vi "Actor Core.vi"(8 "error in":errorcluster, 11 "MQTT-Server in":refnum<class "MQTT-Server.lvclass">) -> (0 "error out":errorcluster, 3 "Actor out":refnum<class "Actor.lvclass">)   [LabVIEW 2023, in "MQTT-Server.lvlib" / "MQTT-Server.lvclass"]
doc: "(<B>Filename</B>: Actor Framework.lvlib:Actor.lvclass:Actor Core.vi)\n\nReceives messages to the actor, reacts to them, and initiates any error handling that may shut the actor down.\n\nDescendant classes may override this VI to append parallel tasks for the actor to complete while it handles messages. Overrides use the Call Parent Class Method node."
uses:
  MQTT-Server.lvclass
  <vilib>/ActorFramework/Actor/Actor.lvclass
  MQTT-Server.lvclass/MQTT-Server.ctl
  <vilib>/G Open Source Project for LabVIEW/MQTT Broker/Server class/Server.lvclass
  C:/Program Files/National Instruments/LabVIEW 2023/vi.lib/LabVIEW Open Source Project/MQTT Connection/MQTT_Base/Base Class/MQTT_Base.lvclass
  <vilib>/LabVIEW Open Source Project/MQTT Connection/MQTT_Base/Base Class/MQTT_Base.lvclass
panel:
  out "Chart":waveform(dbl)[](graph)
  out "NbConnections":u32
  out "Inbound Message":string
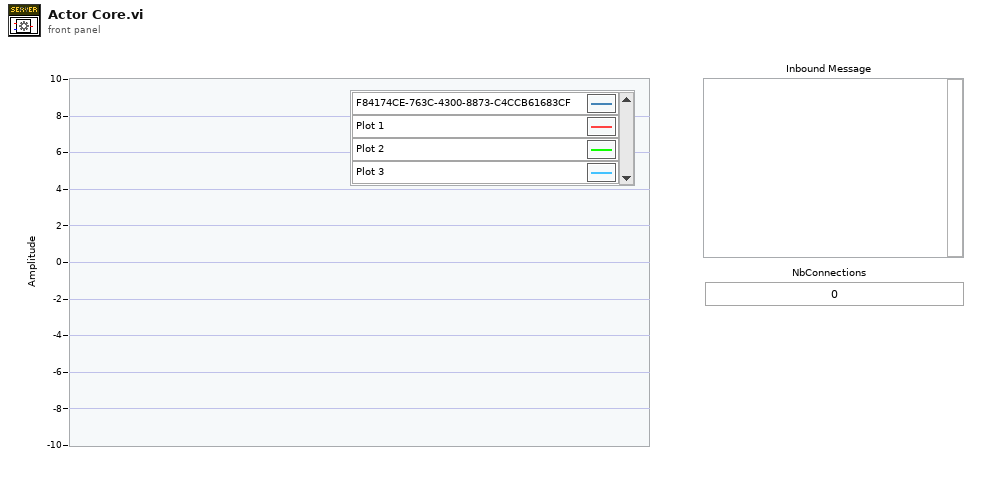
[diagram p1: front panel]
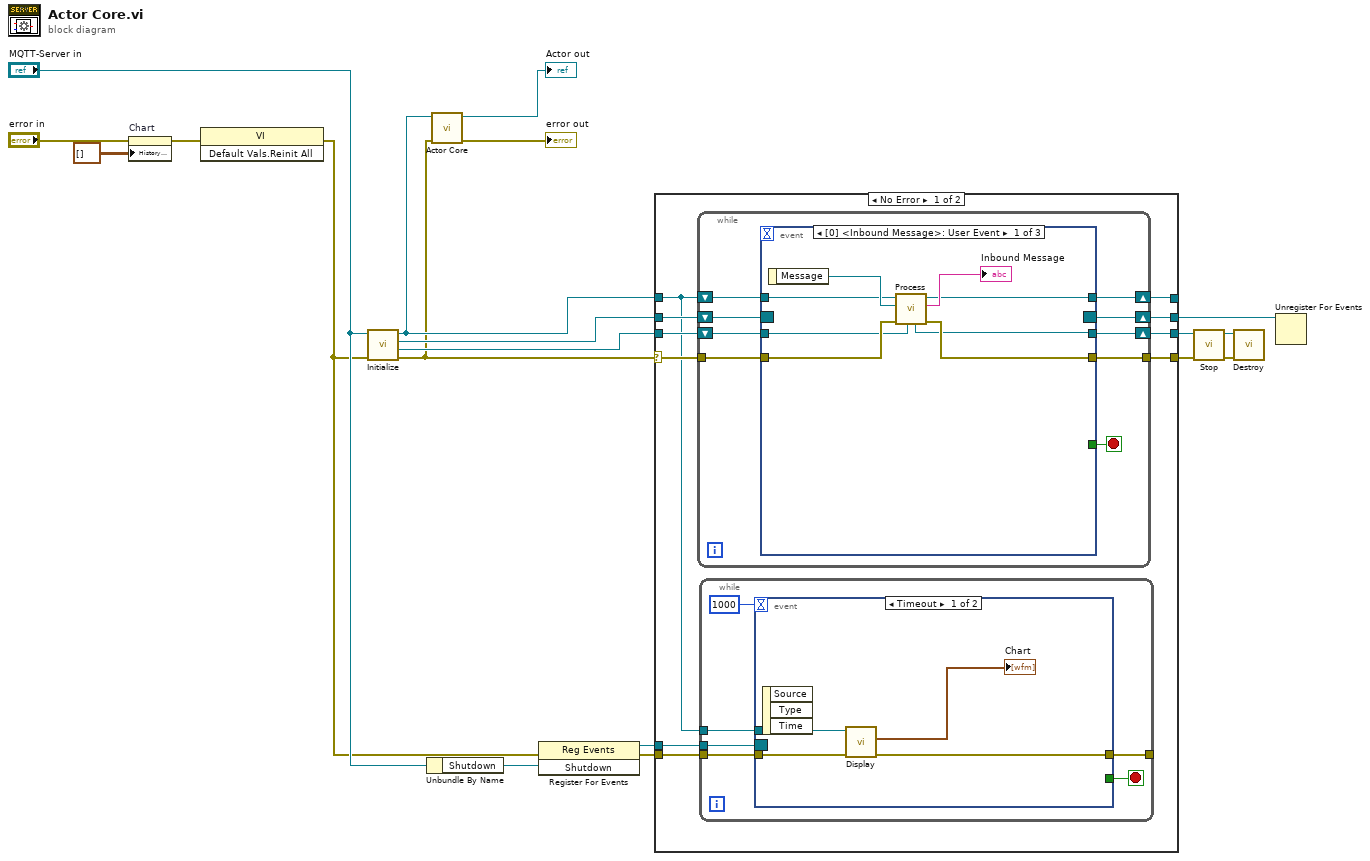
[diagram p0: block diagram]
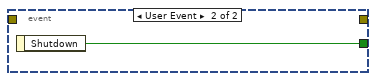
[diagram p2: hidden frame]
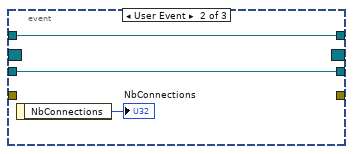
[diagram p3: hidden frame]
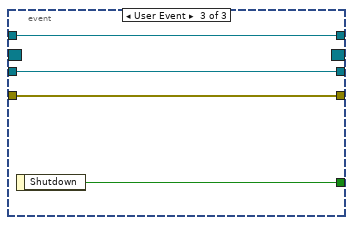
[diagram p4: hidden frame]
diagram:
  n1 = property on="Chart" class="WFChart (strict)"(error in="error in", "History Data"=waveform(dbl)[][] []) -> (error out=w5:errorcluster)  [unwired: 1 in, 1 out]
  n2 = invoke class="VI" method="Default Vals.Reinit All"(error in=w5) -> (error out=w3:errorcluster)  [unwired: 2 in, 2 out]
  n3 = call "Initialize.vi"("error in (no error)"=w3, "MQTT-Server in"="MQTT-Server in") -> ("error out"=w1:errorcluster, "MQTT_Base out"=w11:refnum<class "Server.lvclass">, "Event Ref"=w12:refnum<event-registration>, "MQTT-Server out"=w2:refnum<class "MQTT-Server.lvclass">)  [unwired: 6 in]
  n4 = Unbundle By Name("MQTT-Server in") -> ("Shutdown"=w10:refnum<user-event>)
  n5 = call-parent "Actor Core.vi"("error in"=w1, "Actor in"=w2) -> ("error out"=→"error out":errorcluster, "Actor out"=→"Actor out":refnum<class "Actor.lvclass">)  [unwired: 8 in]
  n6 = register-events(error in=w3, w10) -> (reference out=w8:refnum<event-registration>, error out=w9:errorcluster)  [unwired: 1 in]
  n7 = case shown="No Error" w1 {
    selector: w1 -> [w24 w66]
    tunnel: w11 -> [w29 w68]
    tunnel: [w28 w68] -> w15
    tunnel: w12 -> [w27 w67]
    tunnel: [w26 w67] -> w13
    tunnel: [w25 w66] -> w17
    tunnel: w2 -> [w22 w65]
    tunnel: [w23 w65] -> _
    tunnel: w9 -> [w21 _]
    tunnel: w8 -> [w20 _]
    frame No Error {
      n8 = while {
        shift-right: [w47] -> w28
        shift-left: w29 -> [w49]
        tunnel: [w44] -> w25
        tunnel: w24 -> [w43]
        shift-right: [w45] -> w26
        shift-left: w27 -> [w46]
        shift-right: [w41] -> w23
        shift-left: w22 -> [w42]
        stop <- w48 stop-if-true
        n9 = event shown="[0] <Inbound Message>: User Event" {
          selector: w46 -> [_ _ _]
          dyn-events: [_ _ _] -> w45
          timeout: _ -> [_ _ _]
          tunnel: w49 -> [w52 w60 w64]
          tunnel: [_ _ w62] -> w48
          tunnel: [w51 w60 w64] -> w47
          tunnel: [w54 _ w63] -> w44
          tunnel: w43 -> [w57 _ w63]
          tunnel: w42 -> [w53 w58 w61]
          tunnel: [w50 w58 w61] -> w41
          event User Event {
            n10 = event-data() -> ("Message"=w56:refnum<class "PUBLISH.lvclass">)  [unwired: 1 in]
            n11 = call "Process.vi"("MQTT_Base in"=w52, "error in (no error)"=w57, "Message"=w56, "Server In"=w53) -> ("error out"=w54:errorcluster, "Inbound Message"=→"Inbound Message":string, "Server Out"=w50:refnum<class "MQTT-Server.lvclass">, "MQTT_Base out"=w51:refnum<class "Server.lvclass">)  [unwired: 4 in]
          }
          event User Event {
            n12 = event-data() -> ("NbConnections"=→"NbConnections":u32)  [unwired: 1 in]
          }
          event User Event {
            n13 = event-data() -> ("Shutdown"=w62:bool)  [unwired: 1 in]
          }
        }
      }
      n14 = while {
        tunnel: w22 -> [w33]
        tunnel: w21 -> [w35]
        tunnel: w20 -> [w34]
        tunnel: [w30] -> _
        stop <- w31 stop-if-true
        n15 = event shown="[0] Timeout" {
          selector: w34 -> [_ _]
          dyn-events: _ -> [_ _]
          timeout: 1000 -> [_ _]
          tunnel: w35 -> [w38 _]
          tunnel: w33 -> [w39 _]
          tunnel: [_ w40] -> w31
          tunnel: [w36 _] -> w30
          event Timeout {
            n16 = event-data() -> ()  [unwired: 1 in, 3 out]
            n17 = call "Display.vi"("error in (no error)"=w38, "MQTT-Server in"=w39) -> ("error out"=w36:errorcluster, "Waveform[]"=→"Chart":waveform(dbl)[])  [unwired: 7 in, 1 out]
          }
          event User Event {
            n18 = event-data() -> ("Shutdown"=w40:bool)  [unwired: 1 in]
          }
        }
      }
    }
    frame Error {
    }
  }
  n19 = call <vilib>:"Stop.vi"("error in (no error)"=w17, "MQTT_Base in"=w15) -> ("error out"=w16:errorcluster, "MQTT_Base out"=w14:refnum<class "Server.lvclass">)  [unwired: 7 in, 1 out]
  n20 = call <vilib>:"Destroy.vi"("error in (no error)"=w16, "MQTT_Base in"=w14) -> ()  [unwired: 8 in, 2 out]
  n21 = Unregister For Events(event registration refnum=w13) -> ()  [unwired: 1 in, 1 out]
